vi "MESLog_Cfg_Param.vi"(0 "ItemParamID":string, 1 "DetailResultID":string, 2 "Barcode":string, 3 "BeginDate":string, 4 "EndDate":string, 5 "ParamResType":string, 6 "ParamName":string, 7 "ParamRes1":string, 9 "ParamRes2":string) -> (16 "Cfg_Param":string)   [LabVIEW 2014]
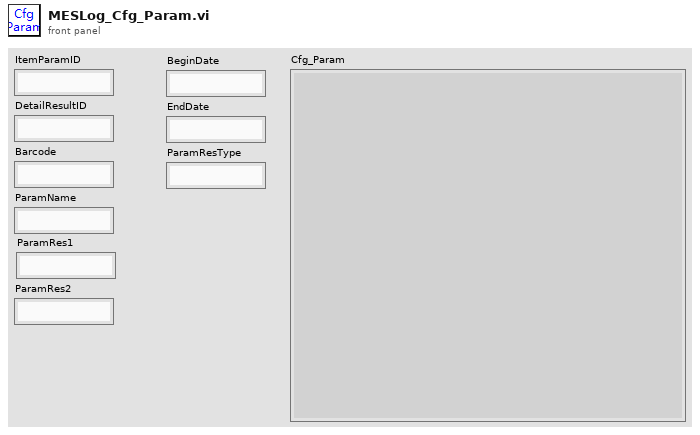
[diagram p1: front panel]
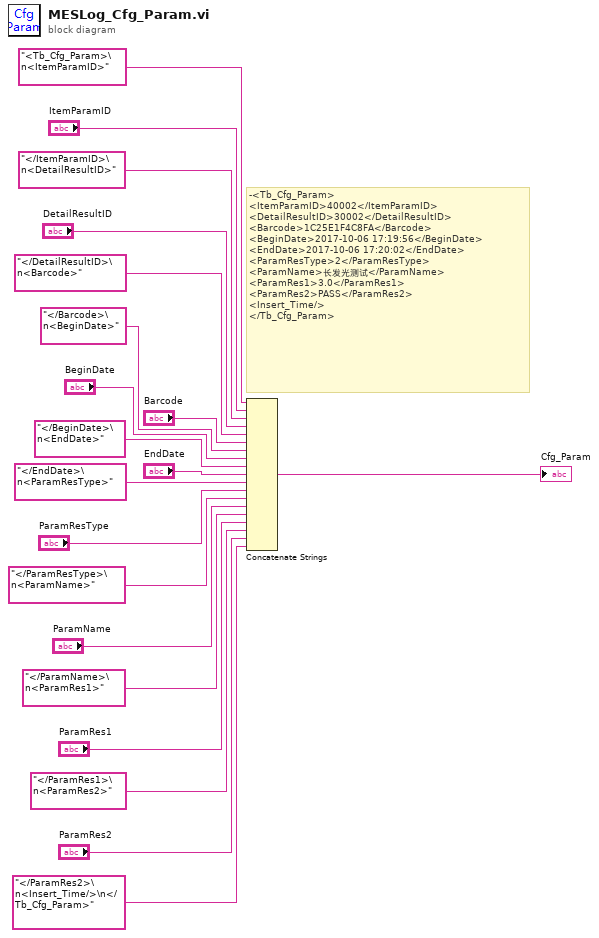
[diagram p0: block diagram]
diagram:
  # "-<Tb_Cfg_Param>\n<ItemParamID>40002</ItemParamID>\n<DetailResultID>30002</DetailResultID>\n<Barcode>1C25E1F4C8FA</Barcode>\n<BeginDate>2017-10-06 17:19:56</BeginDate>\n<EndDate>2017-10-06 17:20:02</EndDate>\n<ParamResType>2</ParamResType>\n<ParamName>长发光测试</ParamName>\n<ParamRes1>3.0</ParamRes1>\n<ParamRes2>PASS</ParamRes2>\n<Insert_Time/>\n</Tb_Cfg_Param>"
  n1 = Concatenate Strings("<Tb_Cfg_Param>\n<ItemParamID>" ("string"), "ItemParamID", "</ItemParamID>\n<DetailResultID>" ("string"), "DetailResultID", "</DetailResultID>\n<Barcode>" ("string"), "Barcode", "</Barcode>\n<BeginDate>" ("string"), "BeginDate", "</BeginDate>\n<EndDate>" ("string"), "EndDate", "</EndDate>\n<ParamResType>" ("string"), "ParamResType", "</ParamResType>\n<ParamName>" ("string"), "ParamName", "</ParamName>\n<ParamRes1>" ("string"), "ParamRes1", "</ParamRes1>\n<ParamRes2>" ("string"), "ParamRes2", "</ParamRes2>\n<Insert_Time/>\n</Tb_Cfg_Param>" ("string")) -> (→"Cfg_Param":string)
